vi "Record Error.vi"(6 "Type":string(combo)="Error", 8 "error in":errorcluster, 11 "Explain":string) -> (0 "error out":errorcluster, 3 "Error string":string)   [LabVIEW 2018]
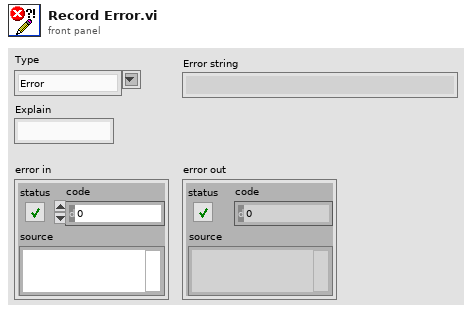
[diagram p1: front panel]
types:
  T1 = enum16{"open", "replace", "create", "open or create", "replace or create", "replace or create with confirmation"}
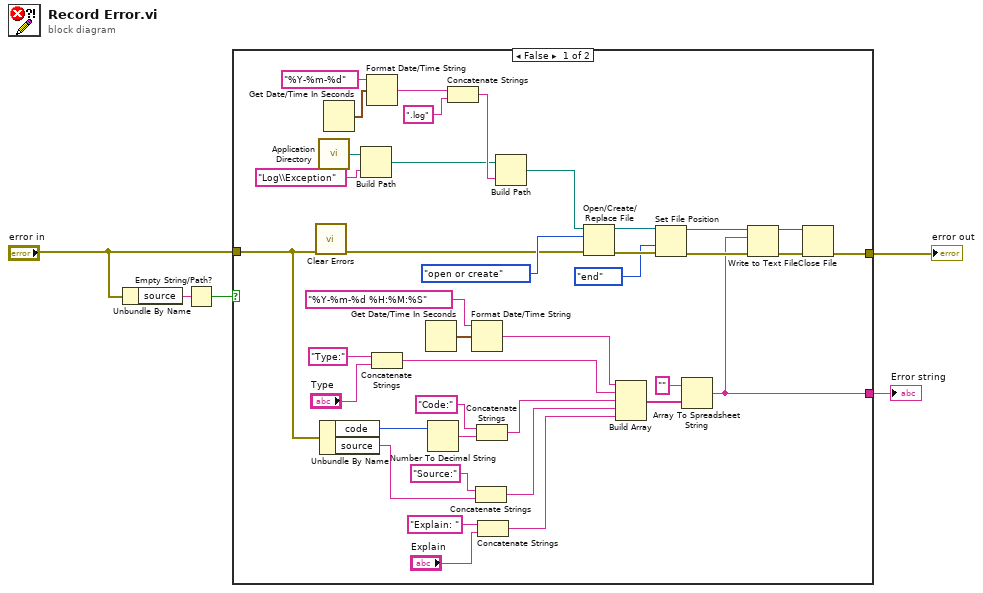
[diagram p0: block diagram]
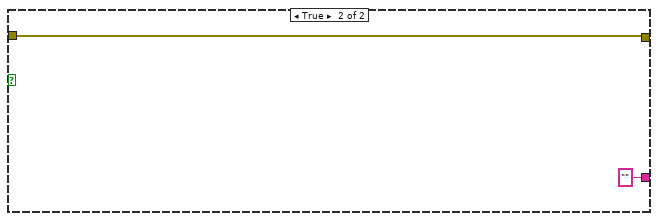
[diagram p2: hidden frame]
diagram:
  n1 = Unbundle By Name("error in") -> ("source"=w5:string)
  n2 = Empty String/Path?(string/path=w5) -> (empty?=w4:bool)
  n3 = case shown="False" w4 {
    tunnel: "error in" -> [w16 w46]
    tunnel: [w11 w46] -> w2
    tunnel: [w8 "" ("spreadsheet string")] -> w1
    frame False {
      n4 = call <vilib>:"Clear Errors.vi"("error in (no error)"=w16) -> ("error out"=w6:errorcluster)  [unwired: 5 in, 1 out]
      n5 = call <vilib>:"Application Directory.vi"() -> ("Application Directory"=w43:path)
      n6 = Unbundle By Name(w16) -> ("code"=w22:i32, "source"=w21:string)
      n7 = Get Date/Time In Seconds() -> (seconds since 1Jan1904=w42:timestamp)
      n8 = Build Path(base path=w43, name or relative path="Log\\Exception") -> (appended path=w7:path)
      n9 = Format Date/Time String(time format string (%c)="%Y-%m-%d", seconds (now)=w42) -> (date/time string=w39:string)  [unwired: 1 in]
      n10 = Concatenate Strings("Type:" ("string"), "Type") -> (w12:string)
      n11 = Get Date/Time In Seconds() -> (seconds since 1Jan1904=w27:timestamp)
      n12 = Number To Decimal String(number=w22) -> (decimal integer string=w26:string)  [unwired: 1 in]
      n13 = Concatenate Strings(w39, ".log" ("string")) -> (w38:string)
      n14 = Format Date/Time String(time format string (%c)="%Y-%m-%d %H:%M:%S", seconds (now)=w27) -> (date/time string=w15:string)  [unwired: 1 in]
      n15 = Concatenate Strings("Source:" ("string"), w21) -> (w20:string)
      n16 = Concatenate Strings("Code:" ("string"), w26) -> (w23:string)
      n17 = Concatenate Strings("Explain: " ("string"), "Explain") -> (w18:string)
      n18 = Build Path(base path=w7, name or relative path=w38) -> (appended path=w37:path)
      n19 = Open/Create/Replace File(file path (use dialog)=w37, error in=w6, operation (0:open)=T1."open or create") -> (refnum out=w36:refnum<file>, error out=w35:errorcluster)  [unwired: 3 in, 1 out]
      n20 = Build Array(w15, w12, w23, w20, w18) -> (w9:string[])
      n21 = Set File Position(refnum=w36, from (0:start)=enum16{"start", "end", "current"}."end", error in=w35) -> (refnum out=w32:refnum<file>, error out=w31:errorcluster)  [unwired: 1 in]
      n22 = Array To Spreadsheet String(array=w9, 3:"" ("format string")) -> (spreadsheet string=w8:string)  [unwired: 1 in]
      n23 = Write to Text File(file (use dialog)=w32, text=w8, error in=w31) -> (refnum out=w29:refnum<file>, error out=w30:errorcluster)  [unwired: 1 in, 1 out]
      n24 = Close File(refnum=w29, error in=w30) -> (error out=w11:errorcluster)  [unwired: 1 out]
    }
    frame True {
    }
  }
  "error out" <- w2
  "Error string" <- w1
